vi "MyRIO_FPGA.vi"() -> ()   [LabVIEW 2019]
uses:
  <vilib>/rvi/Emulation/niFpgaGetClockAttributes.vi
  <vilib>/rvi/Emulation/niFpgaSctlEmulationGetInTimedLoop.vi
  <vilib>/rvi/Emulation/niFpgaEmulationReportErrorSimple.vi
  <vilib>/rvi/eio/common/nirviEmuTemplateMethod_errors.vi
  <vilib>/rvi/interface/RandomDataEmulation/niFpgaRandomDataHandleErrors.vi
  <vilib>/rvi/Emulation/niFpgaCriticalErrorInLSC.vi
  <vilib>/eio/EIONode/EIONode.xnode
  <vilib>/rvi/DataTransferAndStorage/Container/XNode/niFpgaContainer.xnode
  <vilib>/rvi/interface/RandomDataEmulation/nirviRandomDataFpgaReadWriteTemplate.vi
panel:
  in  "timer":u32=1000
  out "appended array":u16[](array[numeric])
  in  "stop":bool
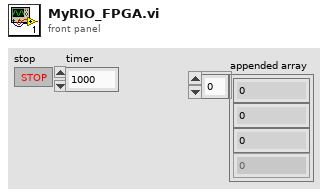
[diagram p1: front panel]
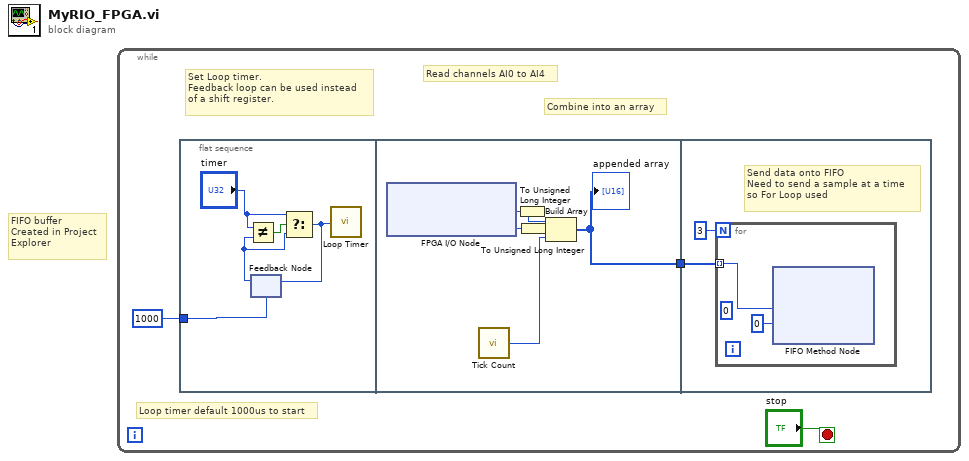
[diagram p0: block diagram]
diagram:
  # "FIFO buffer\nCreated in Project\nExplorer"
  n1 = while {
    stop <- "stop" stop-if-true
    # "Loop timer default 1000us to start"
    # "Combine into an array"
    # "Read channels AI0 to AI4"
    # "Set Loop timer.\nFeedback loop can be used instead\nof a shift register."
    n2 = flat-sequence {
      tunnel: u32 1000 ("Count(uSec)") -> [w8]
      tunnel: [w12] -> w2
      tunnel: w2 -> [w15]
      frame #0 {
        n3 = feedback #1(w8) -> (w5:u32)
        n4 = Not Equal?(x="timer", y=w5) -> (x != y?=w7:bool)
        n5 = Select(t="timer", s=w7, f=w5) -> (s? t:f=w4:u32)
        n6 = feedback-in #1(w4) -> ()
        n7 = call "Loop Timer"("Count(uSec)"=w4) -> ()  [unwired: 1 out]
      }
      frame #1 {
        n8 = xnode "FPGA I/O Node"() -> ("ConnectorC/AI0"=w13:i16, "ConnectorC/AI1"=w14:i16)  [unwired: 2 in, 2 out]
        n9 = call "Tick Count"() -> ("Tick Count(Ticks)"=w9:u32)
        n10 = To Unsigned Long Integer(number=w13) -> (unsigned 32bit integer=w10:u32)
        n11 = To Unsigned Long Integer(number=w14) -> (unsigned 32bit integer=w11:u32)
        n12 = Build Array(w10, w11, w9) -> (w12:u32[])
        "appended array" <- w12
      }
      frame #2 {
        # "Send data onto FIFO\nNeed to send a sample at a time \nso For Loop used"
        n13 = for {
          N: 3 -> [_]
          tunnel: w15 -> [w18] mode=indexing
          (unwired) 0 ("Timeout")
          n14 = xnode ("FIFO Method Node")("Element"=w18, "Timeout"=0) -> ()  [unwired: 1 in, 2 out]
        }
      }
    }
  }
